vi "After Iterative Write.vi"(8 "Error In":errorcluster, 10 "Local":refnum<file>, 11 "SFTP File":refnum<class "SFTP File.lvclass">) -> (0 "Error Out":errorcluster, 2 "Remote Path":string, 3 "SFTP":refnum<class "SFTP.lvclass">)   [LabVIEW 2018, in "Tests.lvlib" / "SFTP File.lvlib"]
uses:
  SFTP File.lvlib
  src/Toolkit/SFTP File/SFTP File.lvclass
  src/Toolkit/SFTP/SFTP.lvclass
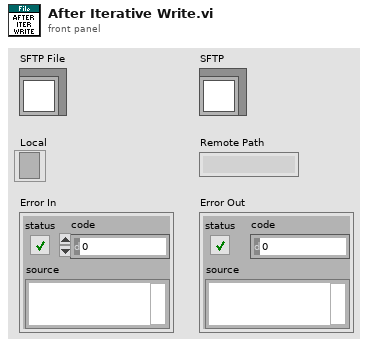
[diagram p1: front panel]
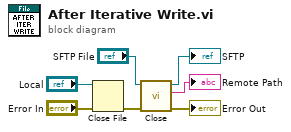
[diagram p0: block diagram]
diagram:
  n1 = Close File(refnum="Local", error in="Error In") -> (error out=w2:errorcluster)  [unwired: 1 out]
  n2 = call "Close.vi"("Error In"=w2, "SFTP File"="SFTP File") -> ("Error Out"=→"Error Out":errorcluster, "Remote Path"=→"Remote Path":string, "SFTP"=→"SFTP":refnum<class "SFTP.lvclass">)  [unwired: 7 in]
